vi "New.vi"(8 "Error In":errorcluster, 11 "Key":string) -> (0 "Error Out":errorcluster, 3 "Escaped Variable":refnum<class "EscapedVariable.lvclass">)   [LabVIEW 2018, in "Toolkit.lvlib" / "Tokens.lvlib" / "EscapedVariable.lvclass"]
uses:
  EscapedVariable.lvclass
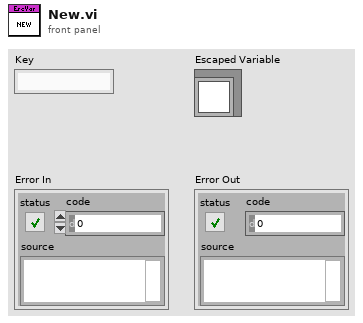
[diagram p1: front panel]
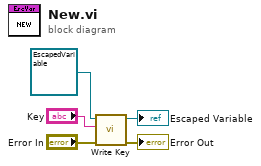
[diagram p0: block diagram]
diagram:
  n1 = call-dynamic "Write Key.vi"("Error In"="Error In", "Key"="Key", "Variable In"=refnum<class "EscapedVariable.lvclass"> refnum ("Mustache.lvlib:Tokens.lvlib:Tag.lvclass")) -> ("Error Out"=→"Error Out":errorcluster, "Variable Out"=→"Escaped Variable":refnum<class "EscapedVariable.lvclass">)  [unwired: 7 in]
